vi "Pre Launch Init.vi"(11 "O3 Frequency Train Actor in":refnum<class "O3 Frequency Train Actor.lvclass">) -> (0 "error out":errorcluster, 3 "O3 Frequency Train Actor out":refnum<class "O3 Frequency Train Actor.lvclass">)   [LabVIEW 2014, in "Calibration.lvlib" / "O3 Frequency Train Actor.lvclass"]
doc: "(<B>Filename</B>: Actor Framework.lvlib:Actor.lvclass:Pre Launch Init.vi)\n\nDefines behavior that occurs after the Launch Nested Actor method is invoked but before the actor's Actor Core method begins running.\n\nBy default, this method does nothing. A descendant class may override it to define behavior."
uses:
  O3 Frequency Train Actor.lvclass
  SuperActor/SuperActor.lvclass/SuperActor.ctl
  O3 Frequency Train Actor.lvclass/O3 Frequency Train Actor.ctl
  SuperActor/Read Log Session.vi
  SuperActor/SuperActor.lvclass
  <userlib>/_Session Fwk/Session - Root.lvclass
  reusable/Session APIs/Session Log/System Log.lvclass
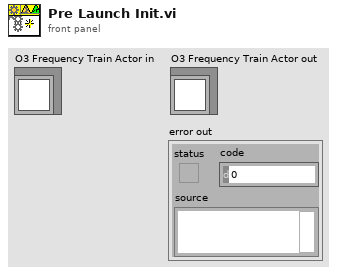
[diagram p1: front panel]
types:
  T1 = typedef "Session - Root.lvclass/Session Handle.ctl" = refnum<data-value>
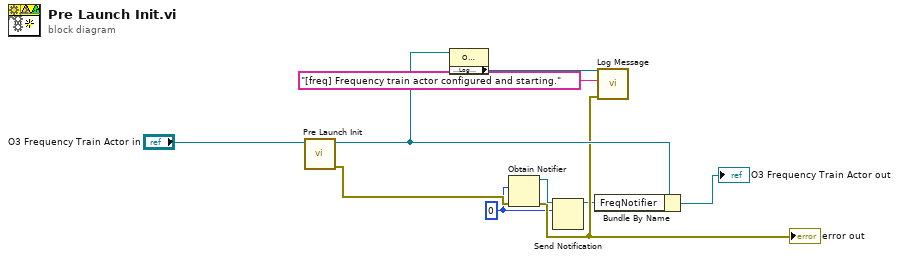
[diagram p0: block diagram]
diagram:
  w1 = i64 0 ("Period")
  n1 = call-parent "Pre Launch Init.vi"("Ex Nested in"="O3 Frequency Train Actor in") -> ("error out"=w3:errorcluster, "Ex Nested out"=w7:refnum<class "O3 Frequency Train Actor.lvclass">)  [unwired: 9 in]
  n2 = property class="O3 Frequency Train Actors"(reference=w7) -> ("Accessors:Log Session"=w5:T1)  [unwired: 1 in, 2 out]
  n3 = Obtain Notifier(notification data type=w1, error in (no error)=w3) -> (notifier out=w8:refnum<notifier>, error out=w6:errorcluster)  [unwired: 2 in, 1 out]
  "error out" <- w6
  n4 = Send Notification(notification=w1, notifier=w8) -> (notifier out=w2:refnum<notifier>)  [unwired: 1 in, 1 out]
  n5 = Bundle By Name(cluster=w7, "FreqNotifier"=w2) -> (→"O3 Frequency Train Actor out":refnum<class "O3 Frequency Train Actor.lvclass">)
  n6 = call "Log Message.vi"("error in"=w6, "MSG In"="[freq] Frequency train actor configured and starting.", "session in"=w5) -> ()  [unwired: 7 in, 2 out]
